vi "Select ring.vi"(8 "error in (no error)":errorcluster, 11 "RSA in":refnum<class "RSA.lvclass">) -> (0 "error out":errorcluster, 2 "Ringnumber":i32, 3 "RSA out":refnum<class "RSA.lvclass">)   [LabVIEW 2012, in "RSA.lvclass"]
uses:
  RSA.lvclass
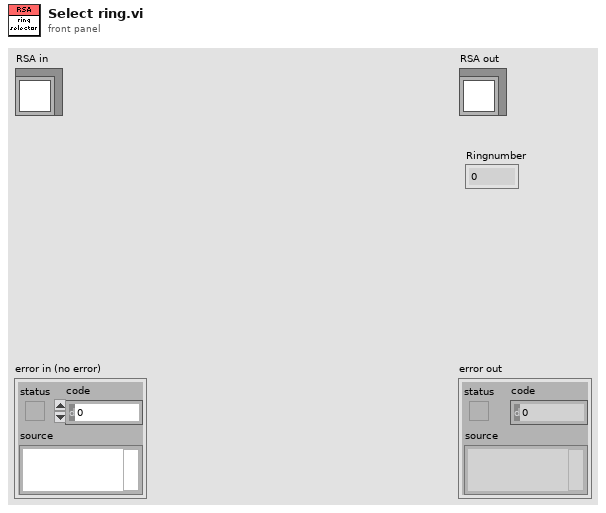
[diagram p1: front panel]
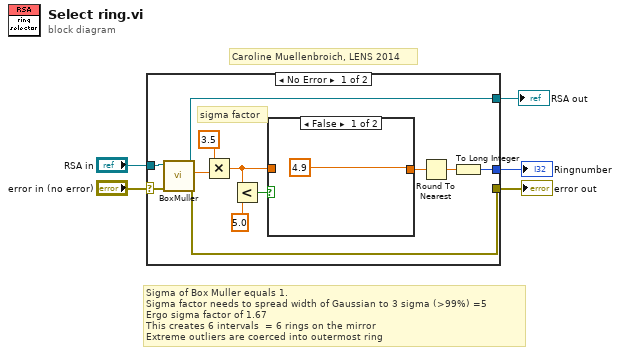
[diagram p0: block diagram]
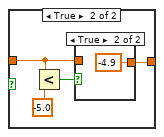
[diagram p2: hidden frame]
diagram:
  # "Caroline Muellenbroich, LENS 2014"
  # "Sigma of Box Muller equals 1. \nSigma factor needs to spread width of Gaussian to 3 sigma (>99%) =5\nErgo sigma factor of 1.67\nThis creates 6 intervals  = 6 rings on the mirror\nExtreme outliers are coerced into outermost ring"
  n1 = case shown="No Error" "error in (no error)" {
    selector: "error in (no error)" -> [w15 w26]
    tunnel: [w17 w26] -> w2
    tunnel: [w13 w25] -> w3
    tunnel: "RSA in" -> [w14 w25]
    tunnel: [w16 _] -> w1
    frame No Error {
      # "sigma factor"
      n2 = call-dynamic "BoxMuller.vi"("error in (no error)"=w15, "RSA in"=w14) -> ("error out"=w17:errorcluster, "random1"=w12:dbl, "RSA out"=w13:refnum<class "RSA.lvclass">)  [unwired: 6 in, 1 out]
      n3 = Multiply(x=3.5, y=w12) -> (x*y=w8:dbl)
      n4 = Less?(x=w8, y=5.0) -> (x < y?=w9:bool)
      n5 = case shown="False" w9 {
        tunnel: w8 -> [_ w20]
        tunnel: [4.9 w19] -> w6
        frame False {
        }
        frame True {
          n6 = Less?(x=w20, y=-5.0) -> (x < y?=w21:bool)
          n7 = case shown="True" w21 {
            tunnel: w20 -> [w23 _]
            tunnel: [w23 -4.9 ("y")] -> w19
            frame False {
            }
            frame True {
            }
          }
        }
      }
      n8 = Round To Nearest(number=w6) -> (nearest integer value=w7:dbl)
      n9 = To Long Integer(number=w7) -> (32bit integer=w16:i32)
    }
    frame Error {
    }
  }
  "RSA out" <- w3
  "error out" <- w2
  "Ringnumber" <- w1
